vi "Build Time Name.vi"(10 "Base File Name":string, 11 "Timestamp":timestamp) -> (2 "Time Name":string)   [LabVIEW 2014, in "TDMS Logger.lvlib" / "TDMS Logger.lvclass"]
uses:
  TDMS Logger.lvclass
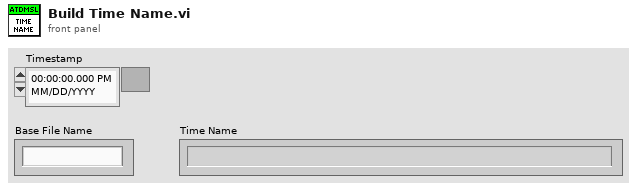
[diagram p1: front panel]
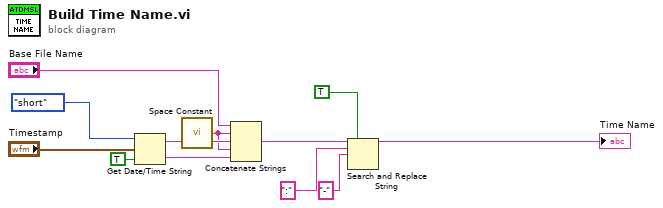
[diagram p0: block diagram]
diagram:
  n1 = Get Date/Time String(date format (0)=enum16{"short", "long", "abbreviated"}."short", seconds (now)="Timestamp", want seconds? (F)=TRUE) -> (date string=w10:string, time string=w9:string)
  n2 = call <vilib>:"Space Constant.vi"() -> ("String"=w2:string)
  n3 = Concatenate Strings("Base File Name", w2, w10, w2, w9) -> (w6:string)
  n4 = Search and Replace String(replace all?=TRUE ("replace all? (F)"), input string=w6, search string=":", replace string="-" ("replace string (\"\")")) -> (result string=→"Time Name":string)  [unwired: 4 in, 3 out]
